vi "SetLvLibPath.vi"(0 "LibReader in":refnum<class "LibReader.lvclass">, 1 "LibPath":path, 2 "LibName":string, 5 "error in (no error)":errorcluster) -> (14 "LibReader out":refnum<class "LibReader.lvclass">, 19 "error out":errorcluster)   [LabVIEW 2014, in "LibReader.lvclass"]
uses:
  <resource>/Framework/Providers/Open_GDS/ClassProviders/LibProvider_BaseClassInterface/LibReader_class/LibReader.lvclass
  <resource>/Framework/Providers/Open_GDS/ClassProviders/LibProvider_BaseClassInterface/LibReader_class/LibReader.lvclass/LibReader.ctl
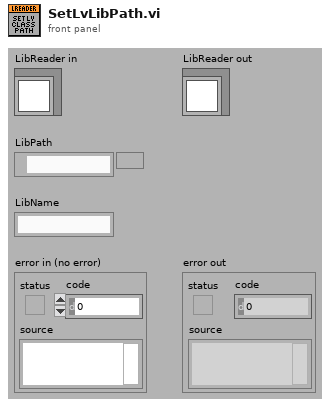
[diagram p1: front panel]
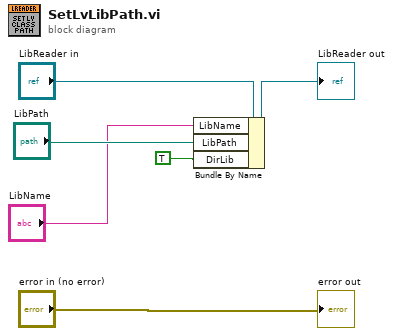
[diagram p0: block diagram]
diagram:
  n1 = Bundle By Name(cluster="LibReader in", "LibName"="LibName", "LibPath"="LibPath", "DirLib"=TRUE ("DirClass")) -> (→"LibReader out":refnum<class "LibReader.lvclass">)
  "error out" <- "error in (no error)"
